vi "rqcBob Read Detection FIFO (PD1).vi"(0 "rqcBob in":refnum<class "rqcBob.lvclass">, 5 "number of elements":u32, 7 "timeout (ms)":i32=100, 11 "error in (no error)":errorcluster) -> (4 "rqcBob out":refnum<class "rqcBob.lvclass">, 6 "Data":u32[](array[numeric]), 10 "Elements Remaining":u32, 15 "error out":errorcluster)   [LabVIEW 2019, in "rqcBob.lvclass"]
uses:
  rqcBob.lvclass
  Custom Controls/rqcBob Main FPGA interface.ctl
  <vilib>/Utility/error.llb/Error Cluster From Error Code.vi
  <vilib>/rvi/errors/niLvFpgaAdjustHostInterfaceError.vi
  <vilib>/rvi/interface/nirviMethod/nirviMethod.xnode
  <vilib>/FPGAPlugInAG/Dynamic/niLvFpga_ReadFifo_Dynamic.vi
  <vilib>/rvi/errors/niLvFpgaMergeErrorWithErrorCode.vi
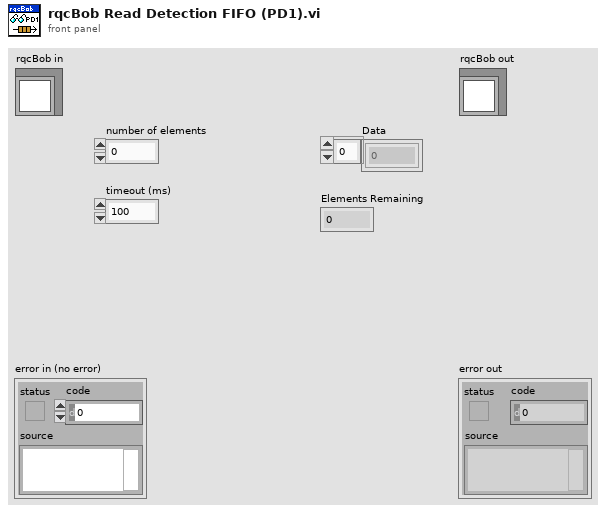
[diagram p1: front panel]
types:
  T1 = typedef "rqcBob.lvclass/rqcBob Main FPGA interface.ctl" = refnum<k20>
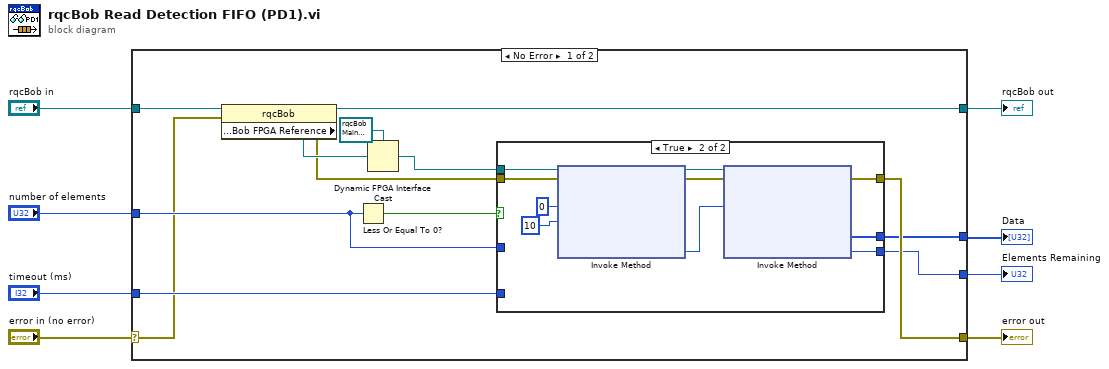
[diagram p0: block diagram]
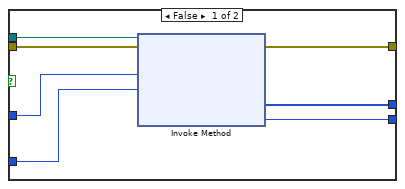
[diagram p2: hidden frame]
diagram:
  n1 = case shown="No Error" "error in (no error)" {
    selector: "error in (no error)" -> [w14 w40]
    tunnel: [w18 w40] -> w7
    tunnel: [w11 w39] -> w5
    tunnel: "rqcBob in" -> [w15 w39]
    tunnel: "number of elements" -> [w20 _]
    tunnel: "timeout (ms)" -> [w19 _]
    tunnel: [w10 _] -> w2
    tunnel: [w9 _] -> w1
    frame No Error {
      n2 = property class="rqcBob"(reference=w15, error in=w14) -> (reference out=w11:refnum<class "rqcBob.lvclass">, error out=w12:errorcluster, "public:Public Properties Access:Bob FPGA Reference"=w16:refnum<k20>)
      n3 = Less Or Equal To 0?(x=w20) -> (x <= 0?=w21:bool)
      n4 = Dynamic FPGA Interface Cast(Session In=T1 refnum ("Bob main FPGA interface"), Type=w16) -> (Session Out=w13:T1)
      n5 = case shown="True" w21 {
        tunnel: w20 -> [w27 _]
        tunnel: [w25 w36] -> w18
        tunnel: w13 -> [w28 w35]
        tunnel: [w26 w33] -> w10
        tunnel: w19 -> [w24 _]
        tunnel: [w23 w30] -> w9
        tunnel: w12 -> [w22 w29]
        frame False {
          n6 = xnode "Invoke Method"("FPGA VI Reference In"=w28, "error in"=w22, "Number of Elements"=w27, "Timeout (ms)"=w24) -> ("error out"=w25:errorcluster, "Data"=w26:u32[], "Elements Remaining"=w23:u32)  [unwired: 1 out]
        }
        frame True {
          n7 = xnode "Invoke Method"("FPGA VI Reference In"=w35, "error in"=w29, "Number of Elements"=u32 0, "Timeout (ms)"=10) -> ("FPGA VI Reference Out"=w38:T1, "error out"=w37:errorcluster, "Elements Remaining"=w32:u32)  [unwired: 1 out]
          n8 = xnode "Invoke Method"("FPGA VI Reference In"=w38, "error in"=w37, "Number of Elements"=w32) -> ("error out"=w36:errorcluster, "Data"=w33:u32[], "Elements Remaining"=w30:u32)  [unwired: 1 in, 1 out]
        }
      }
    }
    frame Error {
    }
  }
  "error out" <- w7
  "rqcBob out" <- w5
  "Data" <- w2
  "Elements Remaining" <- w1
